vi "external clock test.vi"() -> ()   [LabVIEW 2012]
uses:
  <vilib>/eio/EIONode/EIONode.xnode
  <vilib>/Platform/TimedLoop/XDataNode/XDataNode.xnode
  <vilib>/Platform/TimedLoop/XDataNode/nitl_modes.ctl
  <vilib>/Platform/TimedLoop/XDataNode/XDNodeRunTimeDep.lvlib
  <vilib>/Platform/TimedLoop/XDataNode/wakeup.ctl
  <vilib>/Platform/TimedLoop/XDataNode/timing_clust.ctl
  <vilib>/rvi/eio/common/nirviEmuTemplateMethod_errors.vi
  <vilib>/rvi/DataTransferAndStorage/Container/XNode/niFpgaContainer.xnode
  <vilib>/rvi/interface/RandomDataEmulation/nirviRandomDataFpgaReadWriteTemplate.vi
panel:
  in  "Read Channel":T1(ring)
  in  "DO 0":bool
  in  "Start Acquisition":bool
  out "Init Done":bool
  in  "Force Init":bool
  out "DI 1":bool
  out "DI 0":bool
  in  "Sample Clk Source":u8(ring) items=["50 MHz Internal", "Sync Clk", "External Clk In"]
  in  "Num Samples":u32
  # "Digital I/O"
  # "Acquisition"
  # "Status"
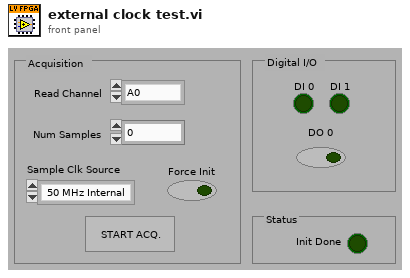
[diagram p1: front panel]
types:
  T1 = enum16{"A0", "A1", "A2", "A3", "A4", "A5", "A6", "A7", "B8", "B9", "B10", "B11", "B12", "B13", "B14", "B15"}
  T2 = typedef "XDNodeRunTimeDep.lvlib/timing_clust.ctl" = cluster{"Expected End [f-1]":u64, "Actual End [f-1]":u64, "Finished Late? [f-1]":bool, "Expected End [i-1]":u64, "Actual End [i-1]":u64, "Finished Late? [i-1]":bool, "Expected Start [i]":u64, "Actual Start [i]":u64, "Expected Start [f]":u64, "Actual Start [f]":u64, "Source Name":string, "Structure Name":string, "Period":i64, "Deadline":i64, "Offset":i64, "Start":i64, "Priority":i32, "Timeout":i32, "Mode":T3, "Wakeup Reason":T4, "Error":errorcluster, "Source Type":string, "Secondary Source Type":string, "Global End Time":u64, "Global Start Time":u64, "Frame Duration":u64, "Iteration Duration":u64, "Assigned CPU":i32, "I/O Scan Engine Mode":u32}
  T3 = typedef "XDNodeRunTimeDep.lvlib/nitl_modes.ctl" = enum32{"No Change", "Process missed periods, maintain original phase", "Discard missed periods, maintain original phase", "Process missed periods, ignore original phase", "Discard missed periods, ignore original phase"}
  T4 = typedef "XDNodeRunTimeDep.lvlib/wakeup.ctl" = enum32{"Normal", "Aborted", "Asynchronous wakeup", "Timing source error", "Timed loop error", "Timeout"}
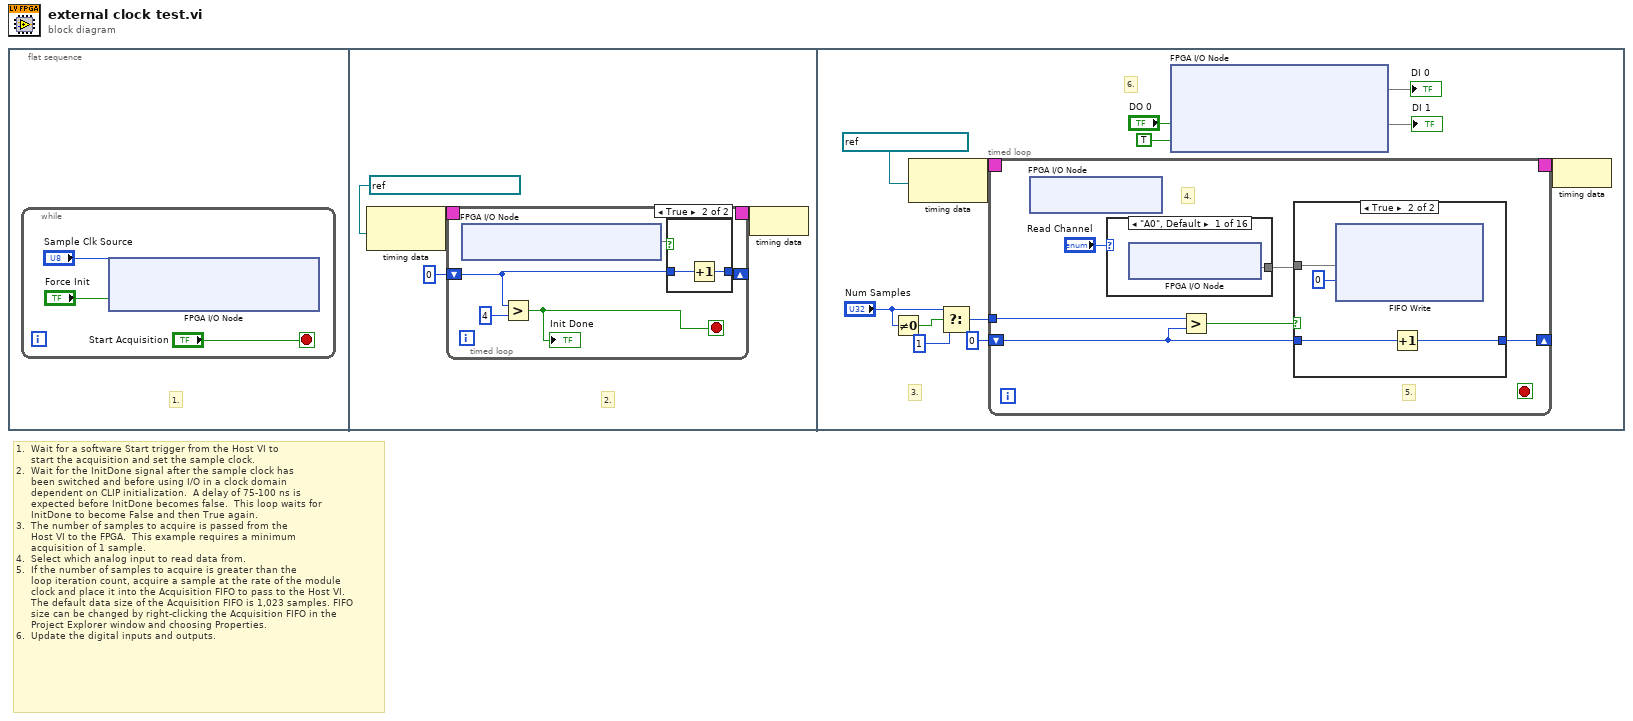
[diagram p0: block diagram]
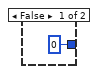
[diagram p2: hidden frame]
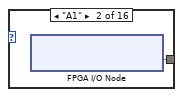
[diagram p3: hidden frame]
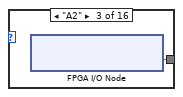
[diagram p4: hidden frame]
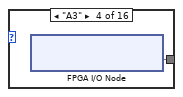
[diagram p5: hidden frame]
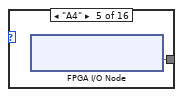
[diagram p6: hidden frame]
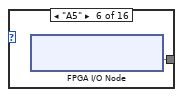
[diagram p7: hidden frame]
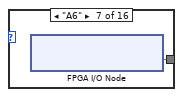
[diagram p8: hidden frame]
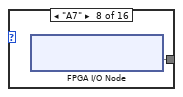
[diagram p9: hidden frame]
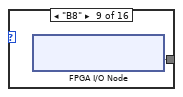
[diagram p10: hidden frame]
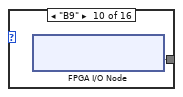
[diagram p11: hidden frame]
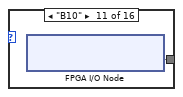
[diagram p12: hidden frame]
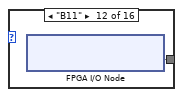
[diagram p13: hidden frame]
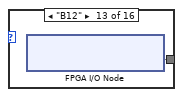
[diagram p14: hidden frame]
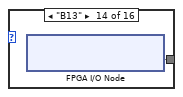
[diagram p15: hidden frame]
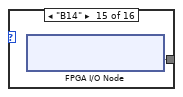
[diagram p16: hidden frame]
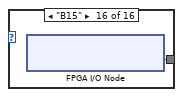
[diagram p17: hidden frame]
diagram:
  # "1.  Wait for a software Start trigger from the Host VI to\n     start the acquisition and set the sample clock.\n2.  Wait for the InitDone signal after the sample clock has \n     been switched and before using I/O in a clock domain \n     dependent on CLIP initialization.  A delay of 75-100 ns is \n     expected before InitDone becomes false.  This loop waits for \n     InitDone to become False and then True again.\n3.  The number of samples to acquire is passed from the \n     Host VI to the FPGA.  This example requires a minimum \n     acquisition of 1 sample.\n4.  Select which analog input to read data from. \n5.  If the number of samples to acquire is greater than the \n     loop iteration count, acquire a sample at the rate of the module \n     clock and place it into the Acquisition FIFO to pass to the Host VI.  \n     The default data size of the Acquisition FIFO is 1,023 samples. FIFO \n     size can be changed by right-clicking the Acquisition FIFO in the \n     Project Explorer window and choosing Properties.\n6.  Update the digital inputs and outputs."
  n1 = flat-sequence {
    frame #0 {
      # "1."
      n2 = while {
        stop <- "Start Acquisition" stop-if-true
        n3 = xnode "FPGA I/O Node"("IO Module\\Sample Clock Select"="Sample Clk Source", "IO Module\\Force Initialization"="Force Init") -> ()  [unwired: 2 in, 2 out]
      }
    }
    frame #1 {
      # "2."
      n4 = node-c288(refnum<k21> "40 MHz Onboard Clock" ("Source Name")) -> (w7:T2)
      n5 = timed-loop {
        shift-right: [w11] -> _
        shift-left: u16 0 -> [w10]
        timing: w7 -> [_]
        timing-out: [_] -> w6
        stop <- w8 stop-if-true
        n6 = xnode "FPGA I/O Node"() -> ("IO Module\\Initialization Done"=w12)  [unwired: 1 in, 1 out]
        n7 = Greater?(x=w10, y=u16 4) -> (0:w8:bool)
        "Init Done" <- w8
        n8 = case shown="True" w12 {
          tunnel: [u16 0 w15] -> w11
          tunnel: w10 -> [_ w14]
          frame False {
          }
          frame True {
            n9 = Increment(x=w14) -> (x+1=w15:u16)
          }
        }
      }
      n10 = node-c288(w6) -> ()
    }
    frame #2 {
      # "6."
      # "3."
      n11 = Not Equal To 0?(x="Num Samples") -> (x != 0?=w30:bool)
      n12 = node-c288(refnum<k21> "IO Module Clock 0" ("Source Name")) -> (w33:T2)
      n13 = Select(t="Num Samples", s=w30, f=u32 1) -> (s? t:f=w27:u32)
      n14 = timed-loop {
        timing: w33 -> [_]
        timing-out: [_] -> w32
        shift-right: [w39] -> _
        shift-left: u32 0 -> [w37]
        tunnel: w27 -> [w36]
        stop <- _ stop-if-true
        # "5."
        # "4."
        n15 = xnode "FPGA I/O Node"() -> ()  [unwired: 1 in, 2 out]
        n16 = case shown="\"A0\", Default" "Read Channel" {
          tunnel: [w40 w41 w42 w43 w44 w45 w46 w47 w48 w49 w50 w51 w52 w53 w54 w55] -> w34
          frame "A0", Default {
            n17 = xnode "FPGA I/O Node"() -> ("IO Module\\AI A0"=w40)  [unwired: 1 in, 1 out]
          }
          frame "A1" {
            n18 = xnode "FPGA I/O Node"() -> ("IO Module\\AI A1"=w41)  [unwired: 1 in, 1 out]
          }
          frame "A2" {
            n19 = xnode "FPGA I/O Node"() -> ("IO Module\\AI A2"=w42)  [unwired: 1 in, 1 out]
          }
          frame "A3" {
            n20 = xnode "FPGA I/O Node"() -> ("IO Module\\AI A3"=w43)  [unwired: 1 in, 1 out]
          }
          frame "A4" {
            n21 = xnode "FPGA I/O Node"() -> ("IO Module\\AI A4"=w44)  [unwired: 1 in, 1 out]
          }
          frame "A5" {
            n22 = xnode "FPGA I/O Node"() -> ("IO Module\\AI A5"=w45)  [unwired: 1 in, 1 out]
          }
          frame "A6" {
            n23 = xnode "FPGA I/O Node"() -> ("IO Module\\AI A6"=w46)  [unwired: 1 in, 1 out]
          }
          frame "A7" {
            n24 = xnode "FPGA I/O Node"() -> ("IO Module\\AI A7"=w47)  [unwired: 1 in, 1 out]
          }
          frame "B8" {
            n25 = xnode "FPGA I/O Node"() -> ("IO Module\\AI B8"=w48)  [unwired: 1 in, 1 out]
          }
          frame "B9" {
            n26 = xnode "FPGA I/O Node"() -> ("IO Module\\AI B9"=w49)  [unwired: 1 in, 1 out]
          }
          frame "B10" {
            n27 = xnode "FPGA I/O Node"() -> ("IO Module\\AI B10"=w50)  [unwired: 1 in, 1 out]
          }
          frame "B11" {
            n28 = xnode "FPGA I/O Node"() -> ("IO Module\\AI B11"=w51)  [unwired: 1 in, 1 out]
          }
          frame "B12" {
            n29 = xnode "FPGA I/O Node"() -> ("IO Module\\AI B12"=w52)  [unwired: 1 in, 1 out]
          }
          frame "B13" {
            n30 = xnode "FPGA I/O Node"() -> ("IO Module\\AI B13"=w53)  [unwired: 1 in, 1 out]
          }
          frame "B14" {
            n31 = xnode "FPGA I/O Node"() -> ("IO Module\\AI B14"=w54)  [unwired: 1 in, 1 out]
          }
          frame "B15" {
            n32 = xnode "FPGA I/O Node"() -> ("IO Module\\AI B15"=w55)  [unwired: 1 in, 1 out]
          }
        }
        n33 = Greater?(x=w36, y=w37) -> (0:w38:bool)
        n34 = case shown="True" w38 {
          tunnel: w34 -> [_ w60]
          tunnel: w37 -> [w56 w58]
          tunnel: [w56 w57] -> w39
          frame False {
          }
          frame True {
            n35 = xnode ("FIFO Write")("Element"=w60, "Timeout"=0) -> ()  [unwired: 1 in, 2 out]
            n36 = Increment(x=w58) -> (x+1=w57:u32)
          }
        }
      }
      n37 = xnode "FPGA I/O Node"("IO Module\\D0 0"="DO 0", "IO Module\\Digital Output Enable"=TRUE ("IO Module\\DigitalOutputEnable")) -> ("IO Module\\DI 0"=→"DI 0", "IO Module\\DI 1"=→"DI 1")  [unwired: 4 in, 4 out]
      n38 = node-c288(w32) -> ()
    }
  }
